vi "Start Sampling and Wait for Finish.vi"(5 "status string ref.":refnum<vi>, 6 "time resolution (0.1 s)":dbl=0.1, 7 "stop button ref.":refnum<vi>, 8 "error in":errorcluster, 10 "timeout":dbl, 11 "instrument handle":refnum<k15>) -> (0 "error out":errorcluster, 2 "timeout exceeded?":bool, 3 "instrument handle out":refnum<k15>)   [LabVIEW 2013, in "varilib.lvlib"]
doc: "Starts sampling of NI SCOPE digitizer, and wait till sampling finished, or timeout was exceeded, or stop button was pressed. Stop button is optional. If reference of string control is wired, a status message with time left till timeout is generated. The time resolution sets the speed of loop, updating of status message or reading of stop button value."
uses:
  varilib.lvlib
  <vilib>/Utility/error.llb/Error Cluster From Error Code.vi
  <vilib>/ErrorRing/Error Ring.xnode
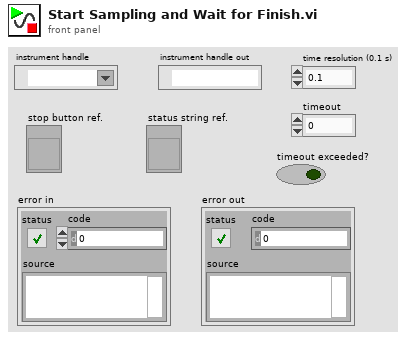
[diagram p1: front panel]
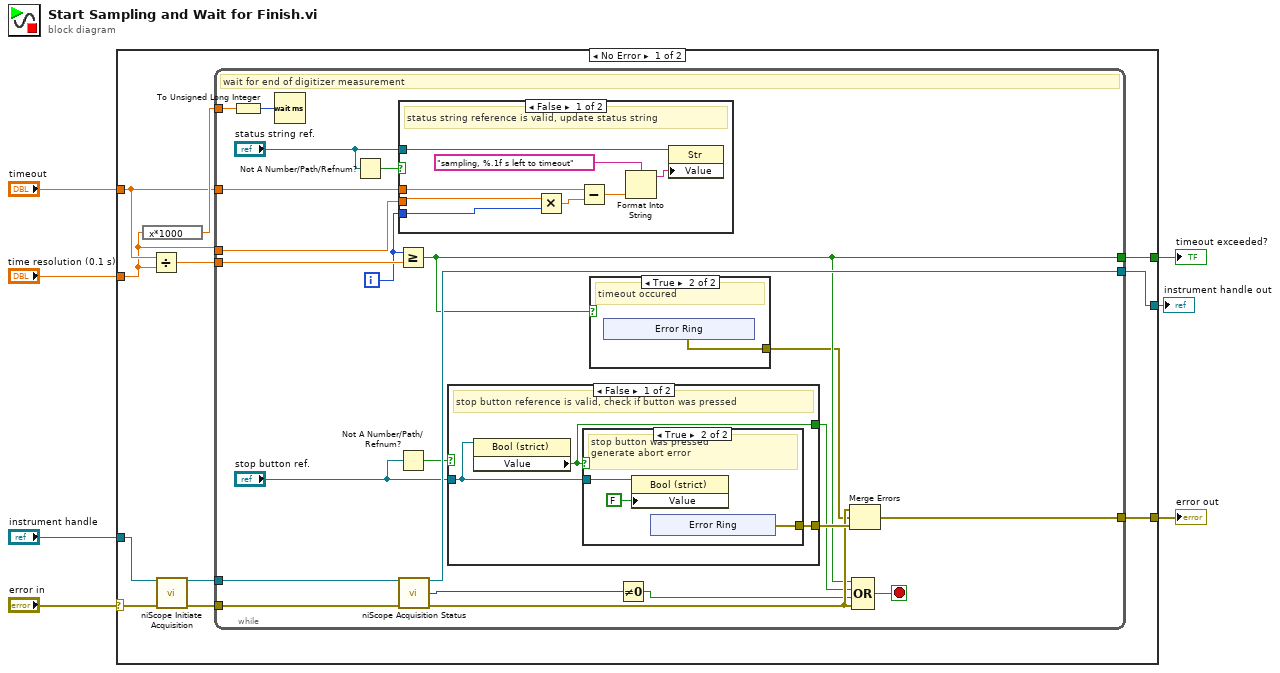
[diagram p0: block diagram]
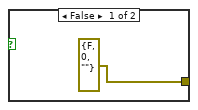
[diagram p2: hidden frame]
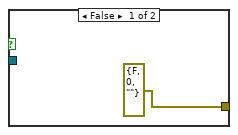
[diagram p3: hidden frame]
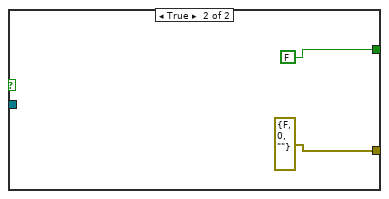
[diagram p4: hidden frame]
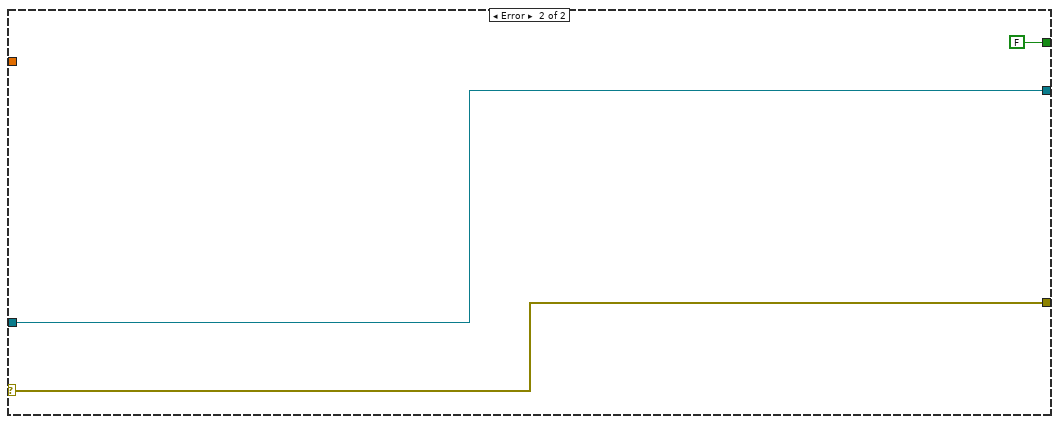
[diagram p6: hidden frame]
diagram:
  n1 = case shown="No Error" "error in" {
    selector: "error in" -> [w10 w72]
    tunnel: [w18 w72] -> w7
    tunnel: [w17 w71] -> w6
    tunnel: [w16 FALSE] -> w5
    tunnel: "instrument handle" -> [w13 w71]
    tunnel: "timeout" -> [w9 _]
    tunnel: "time resolution (0.1 s)" -> [w8 _]
    frame No Error {
      n2 = expression code="x*1000"(w8) -> (w12:dbl)
      n3 = Divide(x=w9, y=w8) -> (x/y=w11:dbl)
      n4 = call <instrlib>:"niScope Initiate Acquisition.vi"("instrument handle"=w13, "error in"=w10) -> ("instrument handle out"=w14:refnum<k15>, "error out"=w15:errorcluster)  [unwired: 12 in]
      n5 = while {
        tunnel: w14 -> [w40]
        tunnel: w15 -> [w39]
        tunnel: [w35] -> w18
        tunnel: [w38] -> w17
        tunnel: [w22] -> w16
        tunnel: w11 -> [w31]
        tunnel: w12 -> [w34]
        tunnel: w9 -> [w32]
        tunnel: w8 -> [w29]
        i -> [w30]
        stop <- w36 stop-if-true
        # "wait for end of digitizer measurement"
        n6 = To Unsigned Long Integer(number=w34) -> (unsigned 32bit integer=w33:u32)
        n7 = Wait (ms)(milliseconds to wait=w33) -> ()  [unwired: 1 out]
        n8 = Not A Number/Path/Refnum?(number/path/refnum="status string ref.") -> (NaN/Path/Refnum?=w25:bool)
        n9 = Greater Or Equal?(x=w30, y=w31) -> (x >= y?=w22:bool)
        n10 = Not A Number/Path/Refnum?(number/path/refnum="stop button ref.") -> (NaN/Path/Refnum?=w23:bool)
        n11 = case shown="False" w25 {
          tunnel: w32 -> [w67 _]
          tunnel: w30 -> [w65 _]
          tunnel: w29 -> [w64 _]
          tunnel: "status string ref." -> [w62 _]
          frame False {
            # "status string reference is valid, update status string"
            n12 = Multiply(x=w64, y=w65) -> (x*y=w63:dbl)
            n13 = Subtract(x=w67, y=w63) -> (x-y=w66:dbl)
            n14 = Format Into String(format string="sampling, %.1f s left to timeout", w66) -> (resulting string=w68:string)  [unwired: 2 in, 1 out]
            n15 = property class="Str"(reference=w62, "Value"=w68) -> ()  [unwired: 1 in, 2 out]
          }
          frame True {
          }
        }
        n16 = call <instrlib>:"niScope Acquisition Status.vi"("instrument handle"=w40, "error in"=w39) -> ("instrument handle out"=w38:refnum<k15>, "acquisition status"=w37:i32, "error out"=w27:errorcluster)  [unwired: 11 in]
        n17 = case shown="False" w23 {
          tunnel: [w50 FALSE ("Value")] -> w19
          tunnel: [w49 errorcluster {"status"=FALSE, "code"=0, "source"=""} ("error out")] -> w28
          tunnel: "stop button ref." -> [w48 _]
          frame False {
            # "stop button reference is valid, check if button was pressed"
            n18 = property class="Bool (strict)"(reference=w48) -> ("Value"=w50:bool)  [unwired: 1 in, 2 out]
            n19 = case shown="True" w50 {
              tunnel: [errorcluster {"status"=FALSE, "code"=0, "source"=""} ("error out") w54] -> w49
              tunnel: w48 -> [_ w52]
              frame False {
              }
              frame True {
                # "stop button was pressed\ngenerate abort error"
                n20 = property class="Bool (strict)"(reference=w52, "Value"=FALSE) -> ()  [unwired: 1 in, 2 out]
                n21 = xnode "Error Ring"() -> ("error out"=w54:errorcluster)
              }
            }
          }
          frame True {
          }
        }
        n22 = case shown="True" w22 {
          tunnel: [errorcluster {"status"=FALSE, "code"=0, "source"=""} ("error out") w42] -> w21
          frame False {
          }
          frame True {
            # "timeout occured"
            n23 = xnode "Error Ring"() -> ("error out"=w42:errorcluster)
          }
        }
        n24 = Not Equal To 0?(x=w37) -> (x != 0?=w20:bool)
        n25 = Merge Errors(w27, w21, w28) -> (w35:errorcluster)
        n26 = Compound Arithmetic op=OR(w22, w19, w20, w27) -> (w36:bool)
      }
    }
    frame Error {
    }
  }
  "error out" <- w7
  "instrument handle out" <- w6
  "timeout exceeded?" <- w5
